vi "Pusher_Client_Global.vi"() -> ()   [LabVIEW 2009, in "Client.lvclass"]
uses:
  Client.lvclass
panel:
  in  "socketID":string
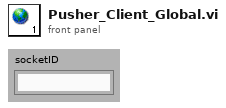
[diagram p1: front panel]
diagram:
